vi "AcquisitionInterface2.vi"() -> ()   [LabVIEW 2025]
uses:
  <vilib>/DAQmx/read.llb/DAQmx Read (Analog 1D Wfm NChan NSamp).vi
  <vilib>/DAQmx/miscellaneous.llb/DAQmx Fill In Error Info.vi
  <vilib>/Waveform/WDTOps.llb/WDT Append Waveforms DBL.vi
panel:
  in  "frequency settings":T1={"frequency (Hz)"=1000.0, "number of samples per cycle"=50.0, "number of cycles"=1.0}
  out "file path out":path
  out "error out":errorcluster
  in  "Save to txt":bool
  in  "stop":bool
  out "data":waveform(dbl)(graph)
  in  "error in":errorcluster
  in  "physical channels":tag
  # "Pulsa este botón para que la señal medida se guarde en un archivo .txt"
  # "La señal se ha guardado en:"
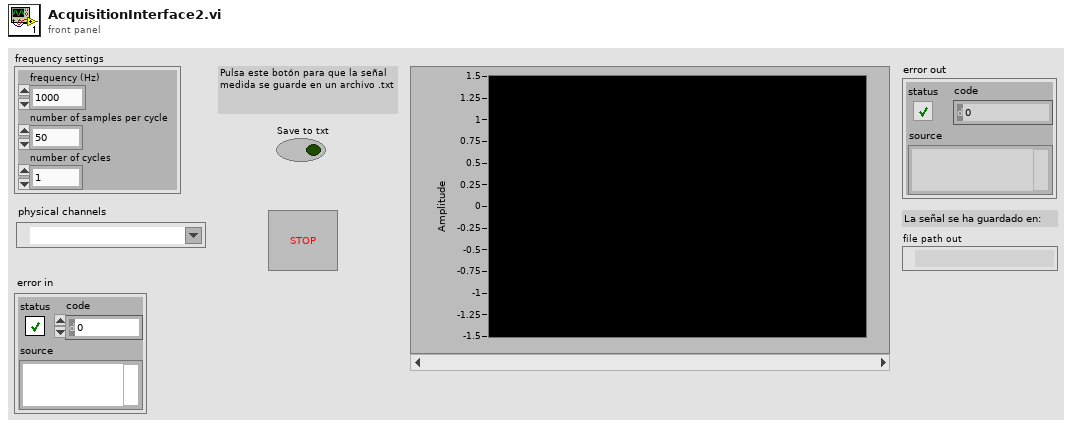
[diagram p1: front panel]
types:
  T1 = cluster{"frequency (Hz)":dbl, "number of samples per cycle":dbl, "number of cycles":dbl}
  T2 = cluster{"units":i32, "input terminal configuration":i32, "maximum value":dbl, "minimum value":dbl}
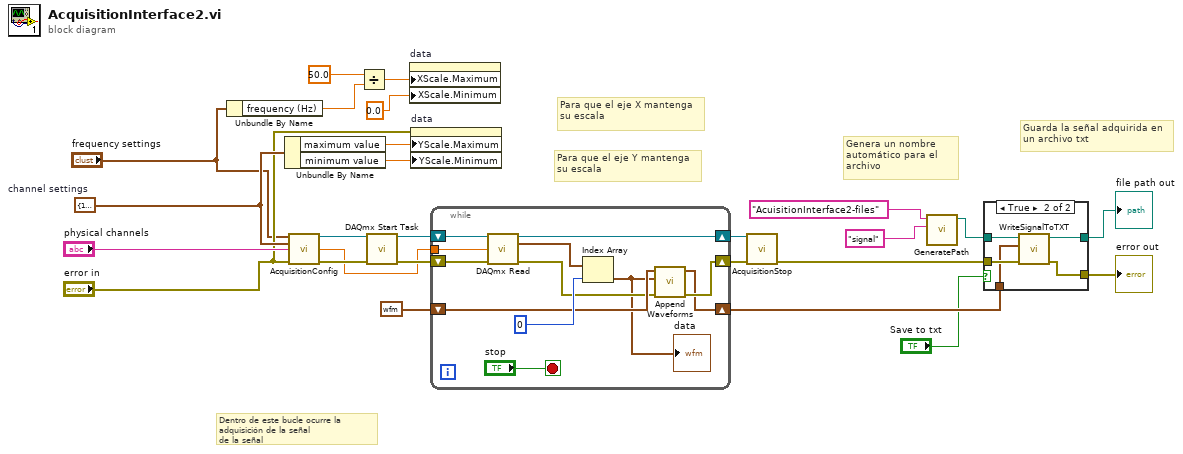
[diagram p0: block diagram]
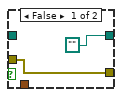
[diagram p2: hidden frame]
diagram:
  w19 = T2 {"units"=10348, "input terminal configuration"=10083, "maximum value"=1.5, "minimum value"=-1.5}  # channel settings
  # "Genera un nombre automático para el archivo"
  # "Para que el eje X mantenga su escala"
  # "Guarda la señal adquirida en\nun archivo txt"
  # "Dentro de este bucle ocurre la adquisición de la señal\nde la señal"
  # "Para que el eje Y mantenga\nsu escala"
  n1 = Unbundle By Name("frequency settings") -> ("frequency (Hz)"=w7:dbl)
  n2 = Unbundle By Name(w19) -> ("maximum value"=w18:dbl, "minimum value"=w17:dbl)
  n3 = call "AcquisitionConfig.vi"("frequency settings"="frequency settings", "channel settings"=w19, "physical channels"="physical channels", "error in"="error in") -> ("task out"=w24:refnum<k21>, "number of samples"=w15:dbl, "error out"=w25:errorcluster)  [unwired: 9 in]
  n4 = Divide(x=50.0, y=w7) -> (x/y=w5:dbl)
  n5 = call <vilib>:"DAQmx Start Task.vi"("task/channels in"=w24, "error in"=w25) -> ("task out"=w22:refnum<k21>, "error out"=w23:errorcluster)  [unwired: 12 in]
  n6 = property on="data" class="WFChart (strict)"("XScale.Maximum"=w5, "XScale.Minimum"=0.0 ("X Scale.Range:Minimum")) -> ()  [unwired: 2 in, 2 out]
  n7 = property on="data" class="WFChart (strict)"(error in="error in", "YScale.Maximum"=w18, "YScale.Minimum"=w17) -> ()  [unwired: 1 in, 2 out]
  n8 = while {
    tunnel: w15 -> [w36]
    shift-right: [w29] -> w21
    shift-left: w23 -> [w30]
    shift-right: [w37] -> w20
    shift-left: w22 -> [w38]
    shift-right: [w27] -> w12
    shift-left: waveform(dbl) {"t0"=timestamp(0 s since 1904-01-01), "dt"=1.0, "Y"=[]} ("waveform out") -> [w32]
    stop <- "stop" stop-if-true
    n9 = call-poly <vilib>:"DAQmx Read.vi"("task/channels in"=w38, "number of samples per channel"=w36, "error in"=w30) -> ("task out"=w37:refnum<k21>, "data"=w33:waveform(dbl)[], "error out"=w31:errorcluster)  [unwired: 10 in]
    n10 = Index Array(array=w33, index=0) -> (element=w28:waveform(dbl))
    "data" <- w28
    n11 = call-poly <vilib>:"Append Waveforms.vi"("error in (no error)"=w31, "waveform B"=w28, "waveform A"=w32) -> ("error out"=w29:errorcluster, "waveform out"=w27:waveform(dbl))  [unwired: 7 in]
  }
  n12 = call "AcquisitionStop.vi"("task/channels in"=w20, "error in"=w21) -> ("error out"=w13:errorcluster)  [unwired: 13 in]
  n13 = call "GeneratePath.vi"("file name (no extension)"="signal", "folder  name"="AcuisitionInterface2-files") -> ("path"=w3:path)  [unwired: 9 in]
  n14 = case shown="True" "Save to txt" {
    tunnel: w13 -> [w40 w45]
    tunnel: w12 -> [_ w44]
    tunnel: [w40 w43] -> w10
    tunnel: [path "" w42] -> w9
    tunnel: w3 -> [_ w41]
    frame False {
    }
    frame True {
      n15 = call "WriteSignalToTXT.vi"("error in"=w45, "waveform"=w44, "file path in"=w41) -> ("error out"=w43:errorcluster, "file path out"=w42:path)  [unwired: 7 in]
    }
  }
  "error out" <- w10
  "file path out" <- w9
